vi "mechanical_action_buttom.vi"() -> ()   [LabVIEW 2019]
panel:
  out "Counter data":u32
  in  "stop":bool
  in  "Mechanical buttom":bool
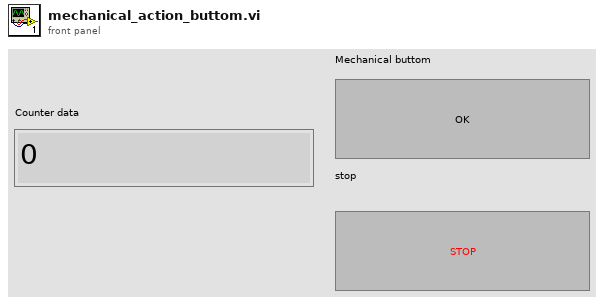
[diagram p1: front panel]
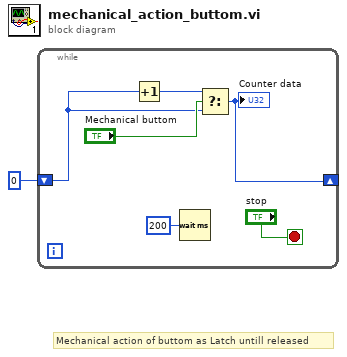
[diagram p0: block diagram]
diagram:
  # "Mechanical action of buttom as Latch untill released"
  n1 = while {
    shift-right: [w6] -> _
    shift-left: u32 0 -> [w4]
    stop <- "stop" stop-if-true
    n2 = Increment(x=w4) -> (x+1=w2:u32)
    n3 = Wait (ms)(milliseconds to wait=u32 200) -> ()  [unwired: 1 out]
    n4 = Select(t=w2, s="Mechanical buttom", f=w4) -> (s? t:f=w6:u32)
    "Counter data" <- w6
  }
